vi "MVE Get Variables In Same Namespace.vi"(8 "error in (no error)":errorcluster, 11 "ProjectItem Refnum":refnum<vi>) -> (0 "error out":errorcluster, 2 "Variable Children":refnum<vi>[](array[refnum]), 3 "dup ProjectItem Refnum":refnum<vi>)   [LabVIEW 2016]
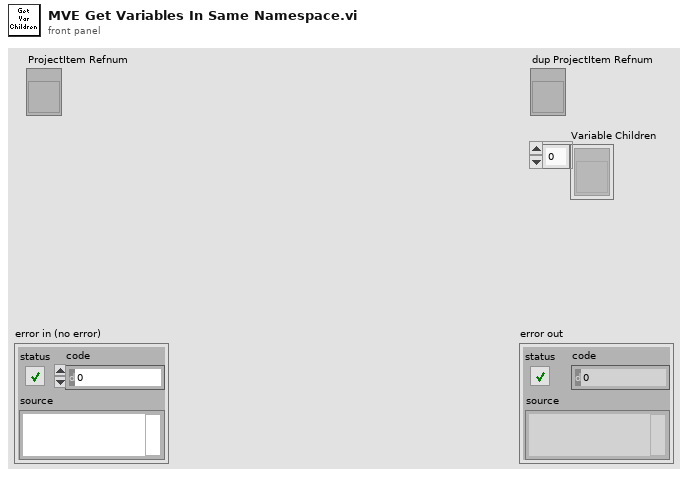
[diagram p1: front panel]
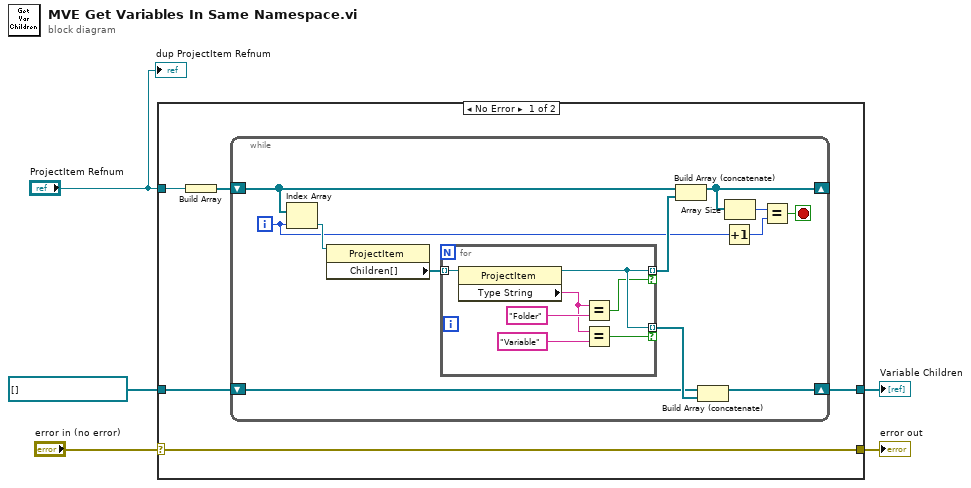
[diagram p0: block diagram]
diagram:
  n1 = case shown="No Error" "error in (no error)" {
    selector: "error in (no error)" -> [w6 w31]
    tunnel: "ProjectItem Refnum" -> [w10 _]
    tunnel: [w8 w30] -> w5
    tunnel: refnum<vi>[] [] -> [w7 w30]
    tunnel: [w6 w31] -> w1
    frame No Error {
      n2 = Build Array(w10) -> (w9:refnum<vi>[])
      n3 = while {
        shift-right: [w17] -> _
        shift-left: w9 -> [w18]
        shift-right: [w14] -> w8
        shift-left: w7 -> [w13]
        i -> [w11]
        stop <- w19 stop-if-true
        n4 = Index Array(array=w18, index=w11) -> (element=w21:refnum<vi>)
        n5 = property class="ProjectItem"(reference=w21) -> ("Children[]"=w22:refnum<vi>[])  [unwired: 1 in, 2 out]
        n6 = for {
          tunnel: w22 -> [w29] mode=indexing
          tunnel: [w27] -> w15 mode=indexing if=w23
          tunnel: [w27] -> w20 mode=indexing if=w26
          n7 = property class="ProjectItem"(reference=w29) -> (reference out=w27:refnum<vi>, "Type String"=w25:string)  [unwired: 1 in, 1 out]
          n8 = Equal?(x=w25, y="Folder") -> (x = y?=w26:bool)
          n9 = Equal?(x=w25, y="Variable") -> (x = y?=w23:bool)
        }
        n10 = Build Array (concatenate)(w18, w20) -> (w17:refnum<vi>[])
        n11 = Build Array (concatenate)(w13, w15) -> (w14:refnum<vi>[])
        n12 = Increment(x=w11) -> (x+1=w12:i32)
        n13 = Array Size(array=w17) -> (size(s)=w16:i32)
        n14 = Equal?(x=w16, y=w12) -> (x = y?=w19:bool)
      }
    }
    frame Error {
    }
  }
  "Variable Children" <- w5
  "error out" <- w1
  "dup ProjectItem Refnum" <- "ProjectItem Refnum"
